vi "Ref Rectangle Selection Window.vi"(8 "error in (no error)":errorcluster) -> (0 "error out":errorcluster, 1 "Error or cancelled":bool)   [LabVIEW 2020]
uses:
  <vilib>/vision/Image Controls.llb/IMAQ Image.ctl
  Typedefs/Channel Selector.ctl
  Typedefs/Ref select window ctrl refs.ctl
  Typedefs/Save-Load enum.ctl
  <vilib>/Utility/miscctls.llb/LVPointTypeDef.ctl
  Globals/gl_Windows Ctrl refs.vi
  Movement Correction/Globals/gl_Movement correction globals.vi
  Global Variables/General Globals.vi
  Global Variables/gl_Images.vi
  Global Variables/gl_UI Ctrl Refs.vi
panel:
  in  "Auto \ncentering\nZ":bool
  in  "Z Ignore":u8=2
  in  "Z Lines":u8=5
  in  "Z pixels":i32=1
  in  "Z Step":i8=2
  out "Ref size":string
  out "Info message":string="Please close this window and run the live imaging mode first to acquire an image"
  out "Tool":i32(ring) items=["None", "Selection Tool", "Point Tool", "Line Tool", "Rectangle Tool", "Oval Tool", "Polygon Tool", "ClosedFreehandTool", "Annulus Tool", "Rotated Rectangle Tool", "Zoom Tool", "Pan Tool", "Polyline Tool", "Freehand Tool"]
  in  "Cancel":bool
  in  "Image intensity":cluster{i16, i16}(slide)={0, 4095} caption="Threshold" scale=0.0..4095.0
  in  "Channel Selector":T1=enum."Green Channel"
  out "AOL Z":dbl format="%#_g um"
  out "AOL Z-Planes":dbl[](array[numeric])
  out "Reference Rectangles":i16[][](array[numeric])
  in  "Full Frame":T2(plugin-control)
  out "Motor Z planes":dbl[](array[numeric])
  out "# of Planes":i32
  out "GreenImageArray":T2[](array[typedef])
  out "RedImageArray":T2[](array[typedef])
  in  "Boundary":i16=2
  in  "OK":bool
  out "Motor Z":dbl format="%#_g um"
  out "Z-Plane":i32 format="Plane %.0f"
  out "Threshold":i16[](array[numeric])
  out "Selected Rectangle":i16[](array[numeric])
  in  "Z-Plane Selector":i32(c297)=7 caption="Z-Plane"
  out "Selection Frame":T2(plugin-control)
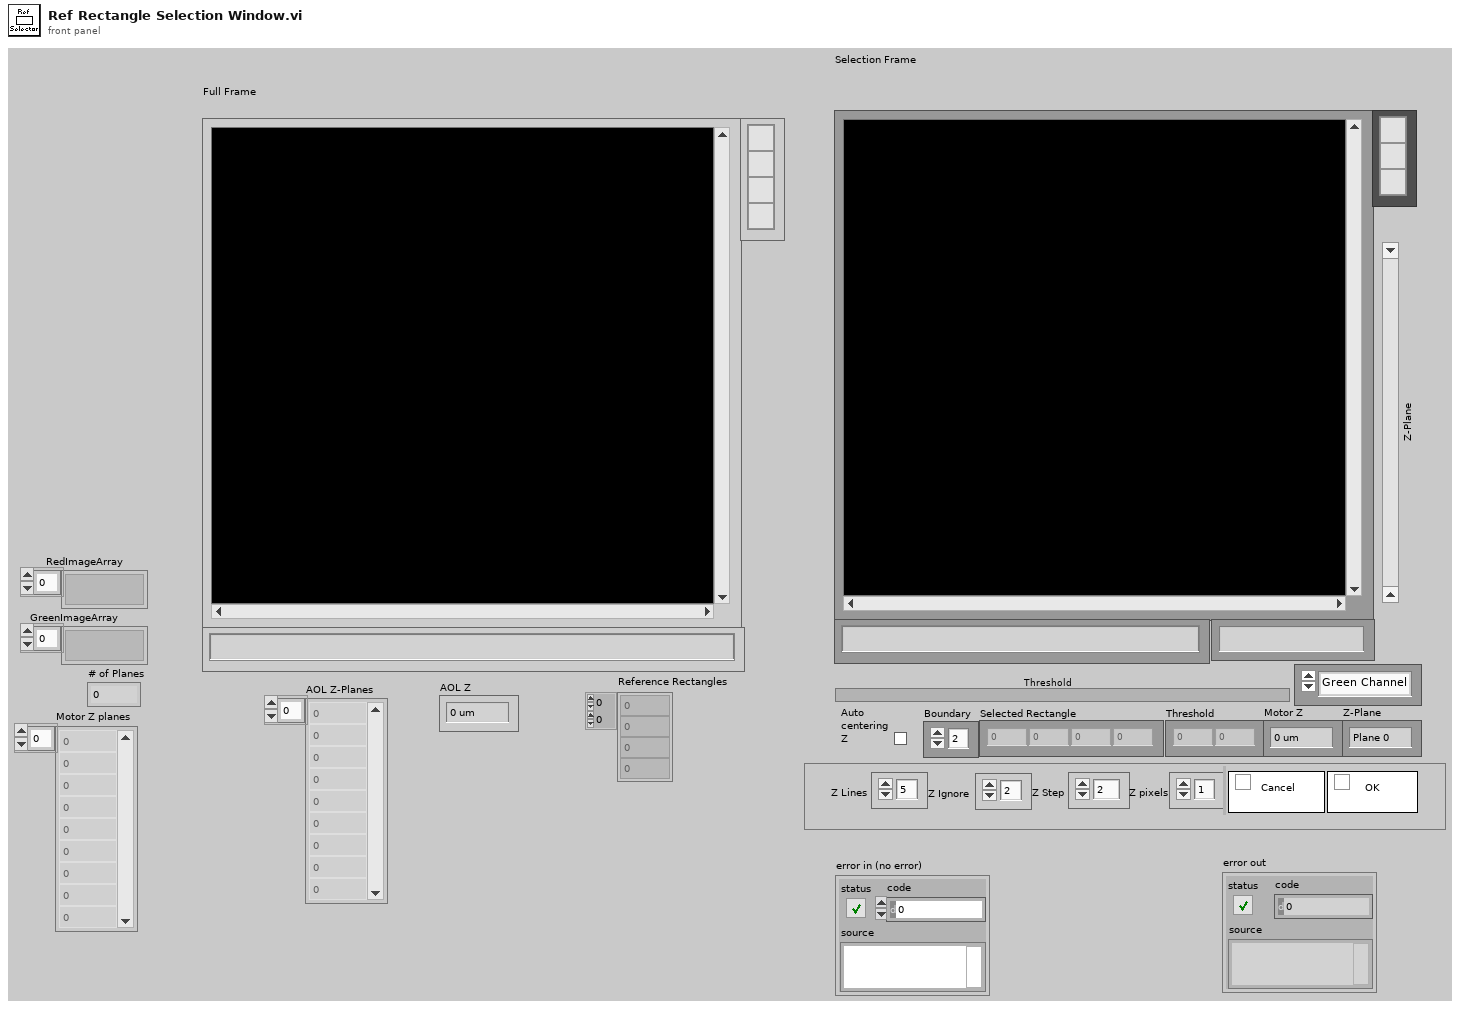
[diagram p1: front panel]
types:
  T1 = typedef "Channel Selector.ctl" = enum16{"Red Channel", "Green Channel", "Blended"}
  T2 = typedef "IMAQ Image.ctl" = refnum<image>
  T3 = typedef "Ref select window ctrl refs.ctl" = cluster{"Channel Selector":refnum<vi>, "Boundary":refnum<vi>, "Image intensity":refnum<vi>}
  T4 = typedef "Save-Load enum.ctl" = enum16{"Save to file", "Load from file", "Compare from file", "Save Backup"}
  T5 = enum16{"Show Binary", "Show Dendrite", "Find Lines"}
  T6 = typedef "LVPointTypeDef.ctl" = cluster{"Horizontal":i16, "Vertical":i16}
  T7 = cluster{"Conversion Method":u32, "Minimum Value":i32, "Maximum Value":i32, "Number Of Shifts":i32}
  T8 = typedef "Reference_Globals.ctl" = cluster{"Refrence data path":path, "Reference Rectangle":i16[][], "AOL Z":dbl, "No of pixels in a miniscan ":i32[], "Threshold":i16[], "No of miniscans":i32[], "Full Frame Size":u16, "Reference Image":T2, "dwelltime":dbl, "Zoom":dbl, "Field of View":dbl, "Z Step":i8, "Z pixels":i32, "Z Lines":u8, "Z Ignore":u8, "Laser":u8, "Auto centering":bool}
  T9 = typedef "AOL_Globals.ctl" = cluster{"Imaging Protocol":T10, "Number of POI":u16, "Number of Miniscans":u16, "Number of Trials":u16, "Number of Cycles ":u64, "# Averaged Frames":u16, "Laser power (%)":u8, "Pockels (V)":dbl, "Acquisition Length (sec)":dbl, "Fill time (us)":dbl, "POI Dwell time (us)":dbl, "Miniscan Dwell time per pixel (us)":dbl, "PMT 1":dbl, "PMT 2":dbl, "Back Apperture (mA)":dbl, "Frame Size":T11, "Center Frequency":dbl, "Field of View (norm)":dbl, "DwellTime (us)":dbl, "Wavelength (nm)":dbl, "Zoom":dbl, "AOL Z":dbl, "AOL Mode":T12, "GridXY":dbl, "GridZ":dbl, "TriggerPeriod (sec)":dbl, "Number of Pixels in Miniscan":u16, "Experiment folder path":path, "X centre":dbl, "Y centre":dbl, "Angle (degrees)":dbl, "Plane Mode":T13, "Threshold":u16[], "Regenerate Chirps":bool, "Rectangle ROI length (pixels)":u16, "Rectangle ROI height (pixels)":u16, "AOD fill":u16, "StartupDelay":i32, "Samples Wait after Trigger":u16, "Slip Cycle":u32, "Add Cycle":bool, "Functional Mode":T14, "Z Start":dbl, "Z Stop":dbl, "# Planes":i32, "Total Pixels":i32, "Variable Miniscan Pixels":u16[], "Use Variable Length":bool, "Use Variable Resolution":bool, "Laser power (%) at Z Start":u8, "Laser power (%) at Z Stop":u8, "Ref Z Step":i8, "Ref Dwell Time (us)":dbl, "Field of View (um)":dbl}
  T10 = typedef "Imaging Protocols enum.ctl" = enum16{"AOL Z-Stack", "Motor Z Stack", "Functional Acquisition", "Single Plane Acquisition", "Volume Acquisition", "Live Imaging", "Live Plane Imaging", "Live Volume Imaging"}
  T11 = typedef "Frame Size.ctl" = u16
  T12 = typedef "AOL modes.ctl" = enum16{"Raster", "Structural", "Pointing", "Mini Scan", "Alignment"}
  T13 = typedef "Plane Mode.ctl" = u16
  T14 = typedef "Functional Mode.ctl" = enum16{"Point", "Line", "Patch", "Plane", "Volume"}
  T15 = typedef "Ref DAQ Param.ctl" = cluster{"Full Frame Size":u16, "Ref Field of View":sgl, "Ref Zoom":i8, "Ref_dwellTime":sgl, "Ref X-pixels-per-line(Npxr)":i16, "Ref Y-lines-per-image(Npyr)":i16, "Ref Z-lines-per-image":i16, "Ignore Z lines":i16, "Ref Scan Cycles":i32, "Ref threshold XY":u16, "Ref threshold Z":u16, "Ref average XY":u16, "Ref Average  Z":u16, "Proportional_scale":fxp<+,16,2>, "Integral_scale":fxp<+/-,16,12>, "Proportional_scale Z":fxp<+,16,2>, "Integral_scale Z":fxp<+/-,16,12>, "Diff_threshold":fxp<+,16,2>, "Diff_threshold _z":fxp<+,16,2>, "Sliding Average":bool, "Ref count reset enabled":bool, "Auto-centering":bool}
  T16 = typedef "UI ctrl refs cluster.ctl" = cluster{"Top level VI path":path, "Top level VI ref":refnum<vi>, "User menu ref":refnum<k9>, "Sub Panel control":refnum<vi>, "Imaging Param Tab":refnum<vi>, "Occurrence-Start drivers":refnum<k4>, "Occurrence-Speed logging initialised":refnum<k4>, "Occurrence-XYZ stage initialised":refnum<k4>, "Exit button":refnum<vi>, "Status ind":refnum<vi>, "Set as origin":refnum<vi>, "Speed Logging":refnum<vi>, "Time Lapse":refnum<vi>, "Live Imaging":refnum<vi>, "AOL Z Stack":refnum<vi>, "Motor Z Stack":refnum<vi>, "Funct Acq button":refnum<vi>, "Hard Shutter":refnum<vi>, "Virtual Shutter":refnum<vi>, "Laser Power":refnum<vi>, "AOL Mode":refnum<vi>, "Frame Size":refnum<vi>, "Field of View":refnum<vi>, "Dwell Time":refnum<vi>, "Zoom":refnum<vi>, "AOL Z":refnum<vi>, "Objective":refnum<vi>, "Axis":refnum<vi>, "Paths & Names":refnum<vi>, "Experiment folder path (ind.)":refnum<vi>, "Last State (Ind.)":refnum<vi>, "Averages":refnum<vi>, "Angle (degrees)":refnum<vi>, "X centre":refnum<vi>, "Y centre":refnum<vi>, "Plane Mode":refnum<vi>, "# Planes":refnum<vi>, "Z Start":refnum<vi>, "Z Stop":refnum<vi>, "Z Step":refnum<vi>, "PMT 1":refnum<vi>, "PMT 2":refnum<vi>, "Stage XYZ Position":refnum<vi>, "Pockels@Z Start":refnum<vi>, "Pockels@Z Stop":refnum<vi>, "Obtain Z Start":refnum<vi>, "Obtain Z Stop":refnum<vi>, "Live stim.trig.period":refnum<vi>, "Live stim.trig.enable":refnum<vi>, "Movement Correction":refnum<vi>, "Load Reference Image":refnum<vi>, "XY Stage Move":refnum<vi>, "MovCor Cluster":refnum<vi>, "RefDAQParam":refnum<vi>, "Funct. Acq. Pockels Modulation":refnum<vi>, "Ref Laser Power":refnum<vi>, "Enable Video Recording":refnum<vi>, "Video Record-Live Imaging":refnum<vi>, "Video Record-Funct acq":refnum<vi>, "Reference Source":refnum<vi>, "AOL Z-stack Chirps Ready (ind)":refnum<vi>, "Target time between mov.cor. ref triggers (ms)":refnum<vi>, "Funct. Acq. Ref frame save":refnum<vi>, "Tracking button":refnum<vi>, "Show ref plots window":refnum<vi>, "Center freq ind (nm)":refnum<vi>, "Pickup mode (ind)":refnum<vi>, "Logging queue (ind)":refnum<vi>, "Back aperture power (ind.)":refnum<vi>, "Power after objective (ind.)":refnum<vi>, "Switch user":refnum<vi>, "Ls1 Conn. Status":refnum<vi>, "Ls1Tuning Status":refnum<vi>, "Ls1 Faults":refnum<vi>, "Ls1 Connection":refnum<vi>, "Ls1 Mode":refnum<vi>, "Ls1 POWER [mW]":refnum<vi>, "Ls1Shutter":refnum<vi>, "Ls1 Wavelength":refnum<vi>, "Ls1 Note":refnum<vi>, "Ls1 Confirm Wav":refnum<vi>, "Ls1 PreChrp Prism1":refnum<vi>, "Ls1 PreChrp Prism2":refnum<vi>, "Ls1 wav top Ind":refnum<vi>, "Ls1 power top Ind":refnum<vi>, "Ls1 Pump peak Hold":refnum<vi>, "Ls1 Status Ind":refnum<vi>, "Ls1 wav cancel":refnum<vi>, "Experiment Type":refnum<vi>, "Biology Information":refnum<vi>, "Camera recording status":refnum<vi>}
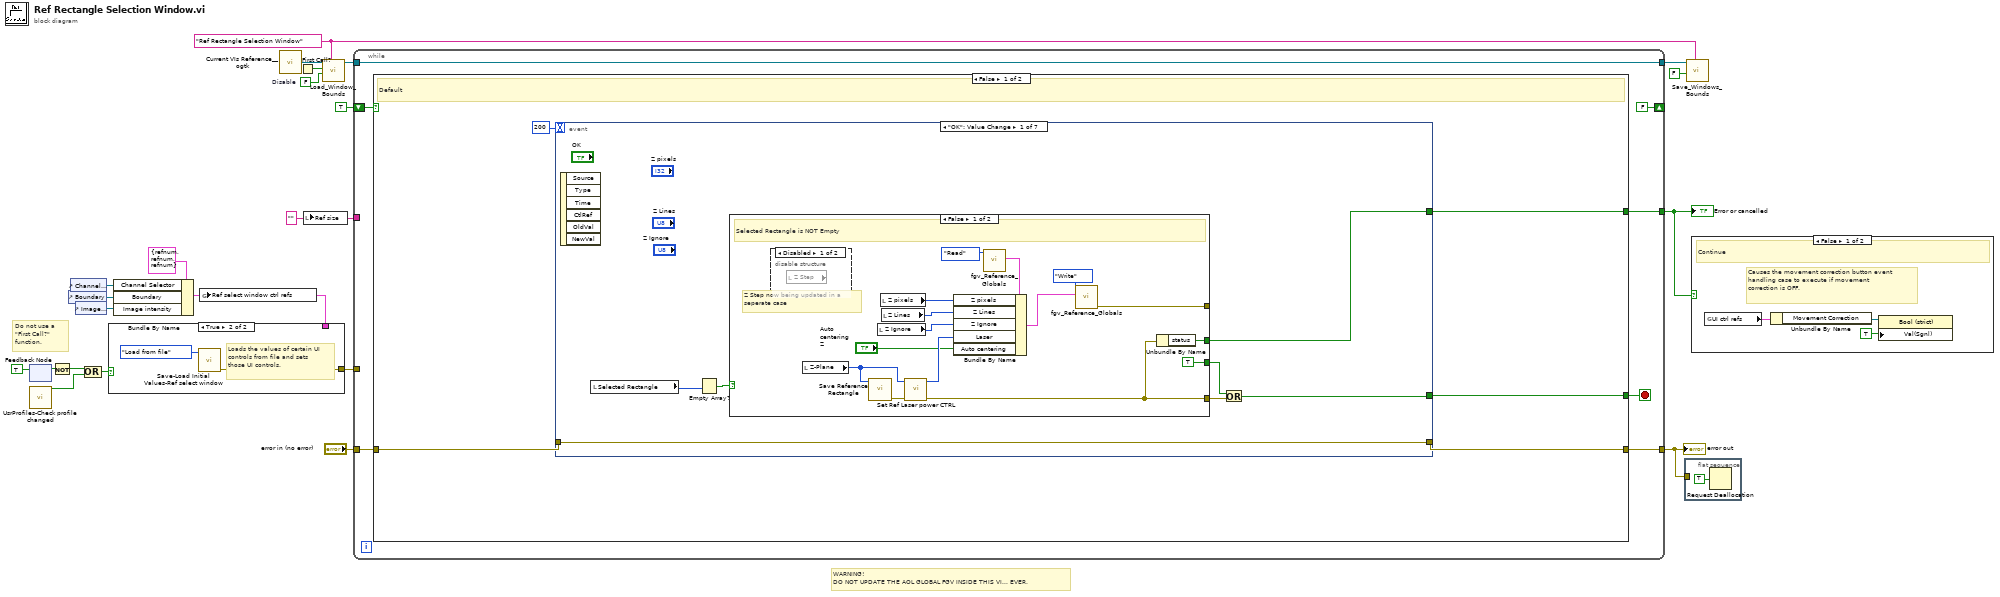
[diagram p0: block diagram]
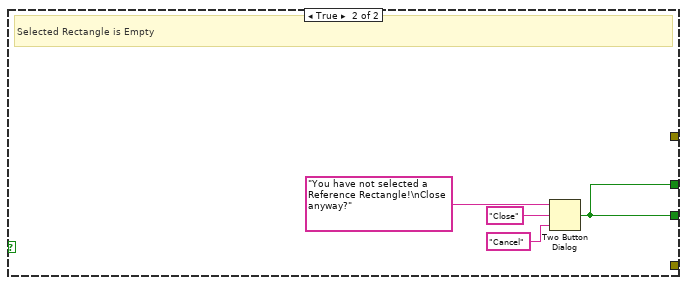
[diagram p5: hidden frame]
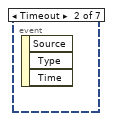
[diagram p6: hidden frame]
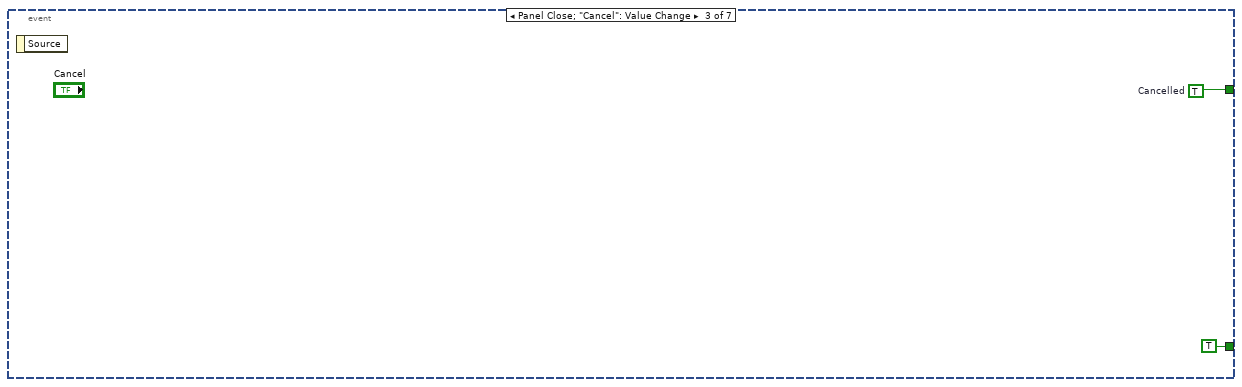
[diagram p7: hidden frame]
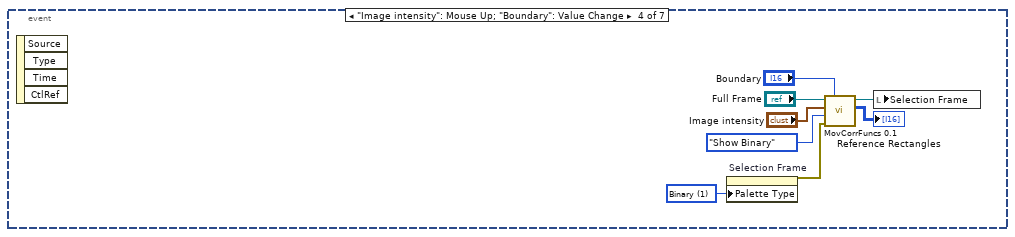
[diagram p8: hidden frame]
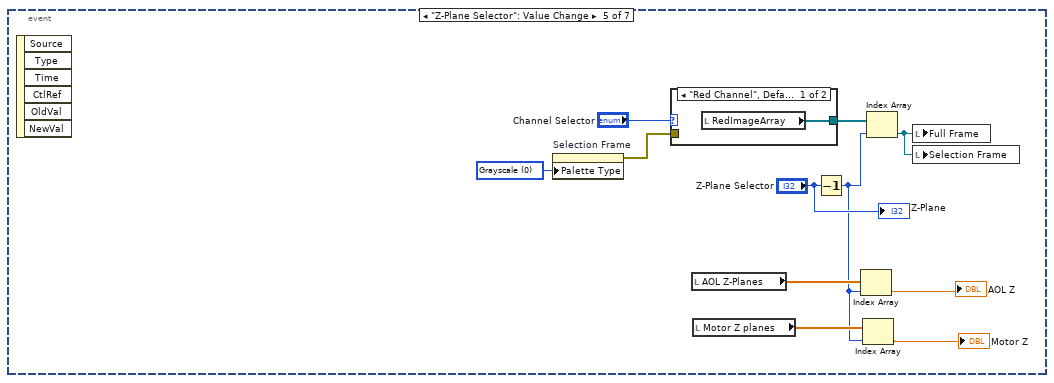
[diagram p9: hidden frame]
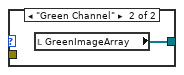
[diagram p10: hidden frame]
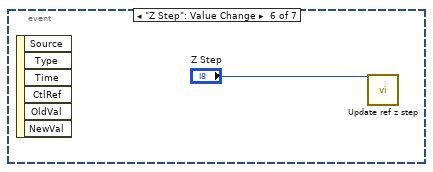
[diagram p11: hidden frame]
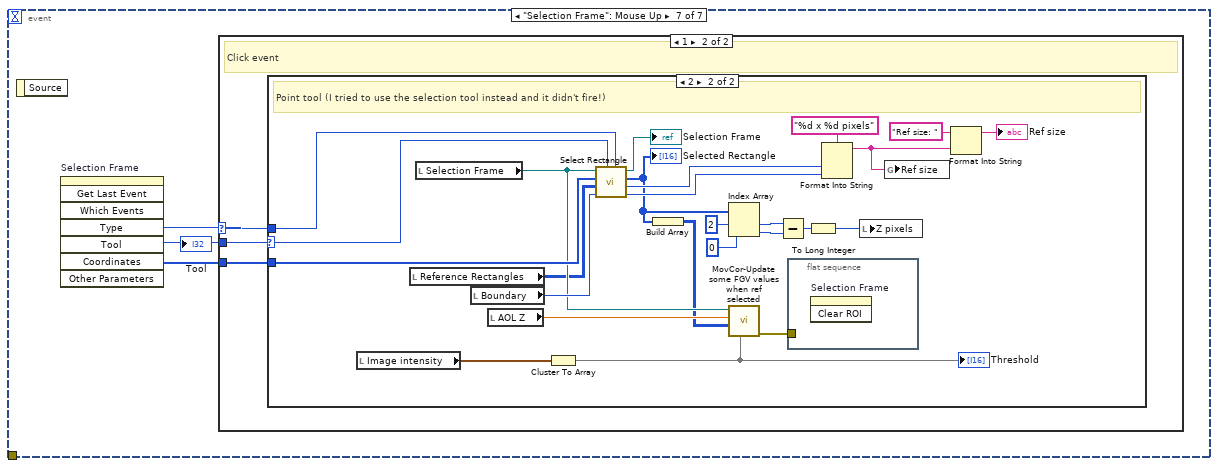
[diagram p12: hidden frame]
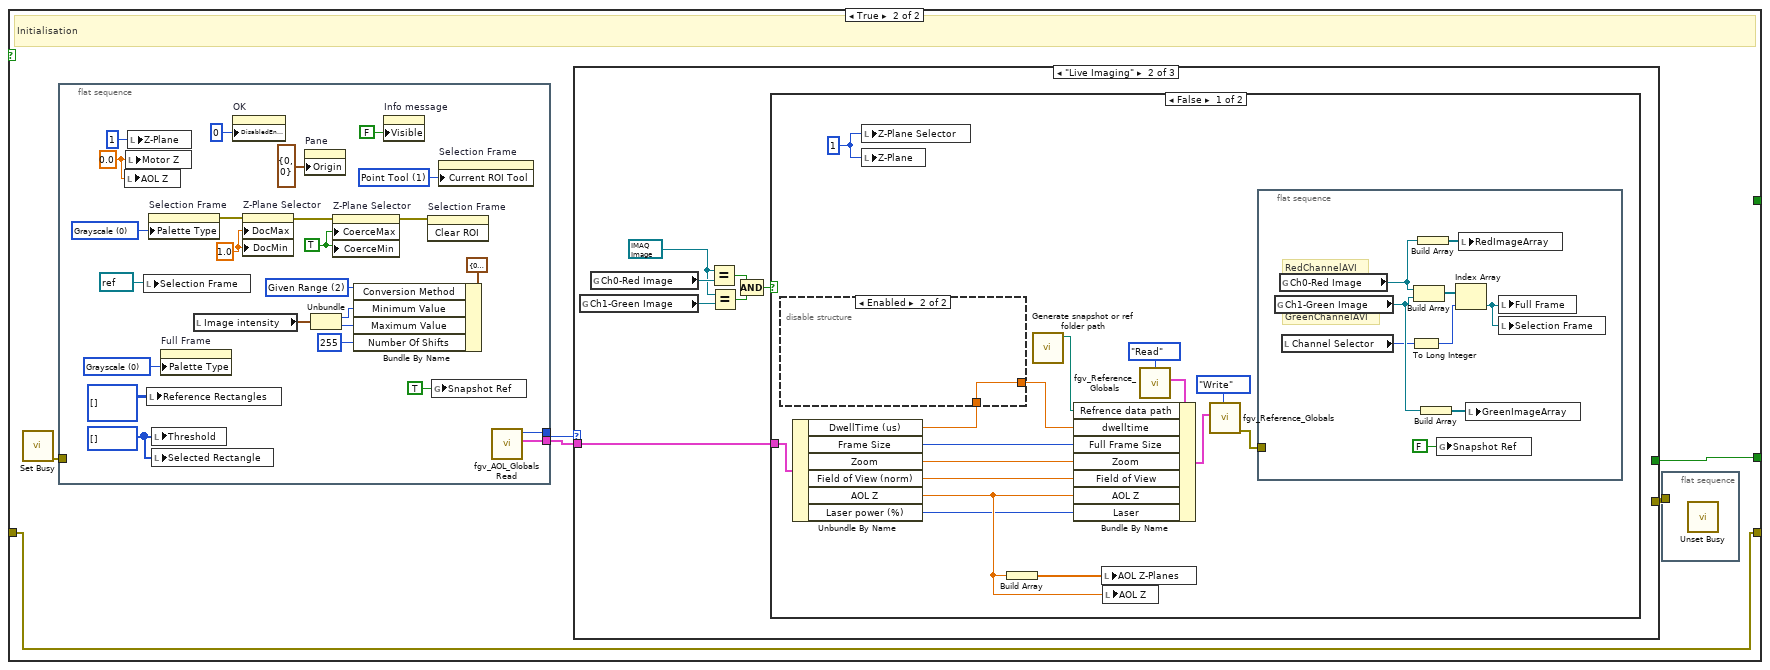
[diagram p15: hidden frame]
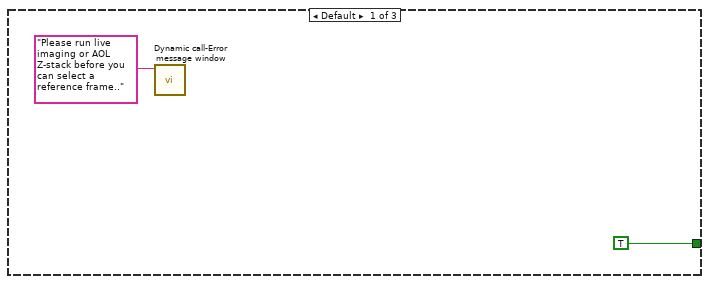
[diagram p16: hidden frame]
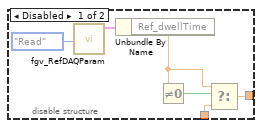
[diagram p17: hidden frame]
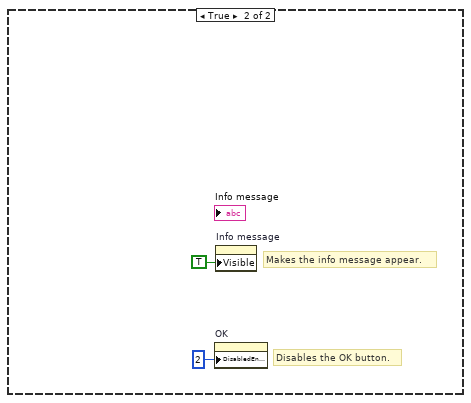
[diagram p18: hidden frame]
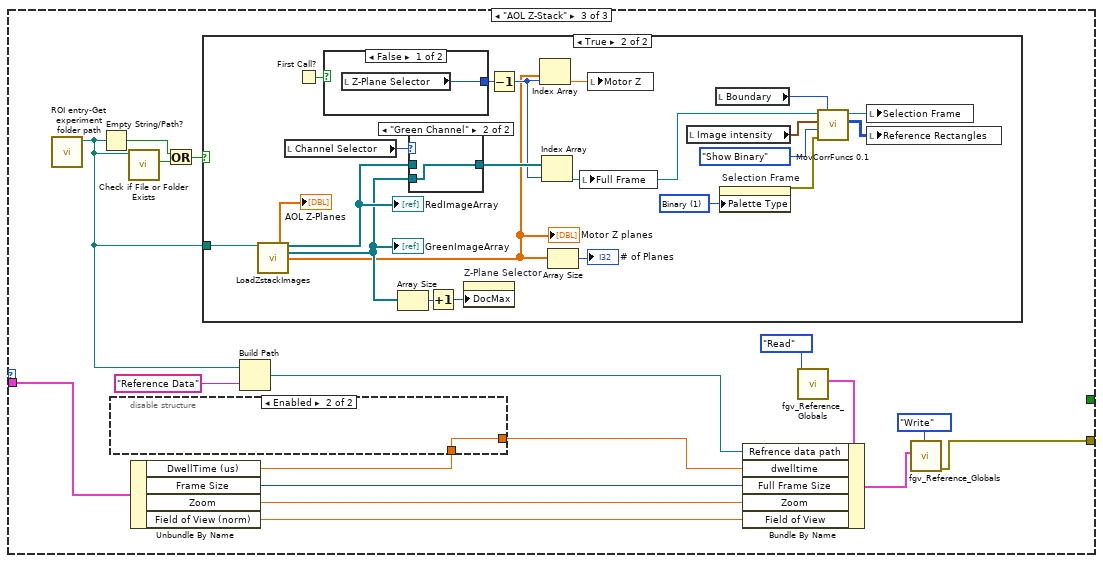
[diagram p19: hidden frame]
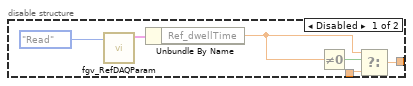
[diagram p20: hidden frame]
diagram:
  w13 = "" ("Ref size")
  w19 = FALSE  # Disable
  w15 = "Ref Rectangle Selection Window" ("Window Name (i.e. Key)")
  # "Do not use a \"First Call?\" function."
  # "WARNING!\nDO NOT UPDATE THE AOL GLOBAL FGV INSIDE THIS VI... EVER."
  n1 = feedback #1() -> (w5:bool)  [unwired: 1 in]
  n2 = feedback-in #1(TRUE) -> ()
  n3 = call "UsrProfiles-Check profile changed.vi"() -> ("Profile changed"=w2:bool)  [unwired: 10 in, 1 out]
  n4 = Not(x=w5) -> (.not. x?=w3:bool)
  n5 = control-ref of="Boundary"() -> (w10:refnum<vi>)
  n6 = control-ref of="Channel Selector"() -> (w11:refnum<vi>)
  n7 = control-ref of="Image intensity"() -> (w9:refnum<vi>)
  n8 = Compound Arithmetic op=OR(w3, w2) -> (w1:bool)
  n9 = Bundle By Name(cluster=T3 {"Channel Selector"=refnum, "Boundary"=refnum, "Image intensity"=refnum} ("Ref select window ctrl refs"), "Channel Selector"=w11, "Boundary"=w10, "Image intensity"=w9) -> (w7:T3)
  n10 = case shown="True" w1 {
    tunnel: [_ w24] -> w6
    tunnel: w7 -> [_ _]
    frame False {
    }
    frame True {
      # "Loads the values of certain UI controls from file and sets those UI controls."
      n11 = call "Save-Load Initial Values-Ref select window.vi"("Function"=Save-Load_enum."Load from file") -> ("error out"=w24:errorcluster)  [unwired: 10 in]
    }
  }
  n12 = global write "gl_Windows Ctrl refs.vi" "Ref select window ctrl refs"(w7) -> ()
  n13 = call <userlib>:"Current VIs Reference__ogtk.vi"() -> ("Current VI's reference"=w21:refnum<vi>)  [unwired: 5 in]
  n14 = First Call?() -> (First Call?: T/F=w20:bool)
  n15 = local write "Ref size"(w13) -> ()
  n16 = call "Load_Window_Bounds.vi"("Window Name (i.e. Key)"=w15, "Disable"=w19, "First Call"=w20, "Window VI's Ref"=w21) -> ("reference out"=w17:refnum<vi>)  [unwired: 4 in, 3 out]
  n17 = while {
    shift-right: [FALSE] -> _
    shift-left: TRUE -> [w30]
    tunnel: "error in (no error)" -> [w29]
    tunnel: [w28] -> w12
    tunnel: [w27] -> w14
    tunnel: [w26] -> w16
    tunnel: w17 -> [w26]
    tunnel: w13 -> [_]
    tunnel: w6 -> [_]
    stop <- w32 stop-if-true
    n18 = case shown="False" w30 {
      tunnel: [w36 w122] -> w32
      tunnel: w29 -> [w35 w119]
      tunnel: [w34 w119] -> w28
      tunnel: [w33 _] -> w27
      frame False {
        # "Default"
        n19 = event shown="[0] \"OK\": Value Change" {
          selector: _ -> [_ _ _ _ _ _ _]
          dyn-events: _ -> [_ _ _ _ _ _ _]
          timeout: 200 -> [_ _ _ _ _ _ _]
          tunnel: [w42 _ TRUE _ _ _ _] -> w36
          tunnel: w35 -> [w43 _ _ _ _ _ _]
          tunnel: [w43 _ _ _ _ _ _] -> w34
          tunnel: [w38 _ w64 _ _ _ _] -> w33
          event "OK": Value Change {
            n20 = event-data() -> ()  [unwired: 1 in, 6 out]
            n21 = local read "Selected Rectangle"() -> (w41:i16[])
            n22 = Empty Array?(array=w41) -> (empty?=w40:bool)
            n23 = case shown="False" w40 {
              tunnel: [TRUE ("T button?") w62] -> w39
              tunnel: [w55 _] -> w44
              tunnel: [w58 w62] -> w38
              tunnel: [w52 _] -> _
              frame False {
                # "Z Step now being updated in a\nseperate case"
                # "Selected Rectangle is NOT Empty"
                n24 = disable-structure shown="Disabled" {
                  frame Disabled {
                    n25 = local read "Z Step"() -> ()  [unwired: 1 out]
                  }
                  frame Enabled {
                  }
                }
                n26 = local read "Z-Plane"() -> (w56:i32)
                n27 = call "Save Reference Rectangle.vi"("Z-Plane"=w56) -> ("error out"=w57:errorcluster)  [unwired: 10 in]
                n28 = local read "Z Ignore"() -> (w46:u8)
                n29 = local read "Z pixels"() -> (w49:i32)
                n30 = local read "Z Lines"() -> (w48:u8)
                n31 = call "Set Ref Laser power CTRL.vi"("error in (no error)"=w57, "Z-Plane"=w56) -> ("error out"=w55:errorcluster, "Laser power (%)"=w47:u8)  [unwired: 8 in]
                n32 = call "fgv_Reference_Globals.vi"("Function"=enum16{"Intialize", "Write", "Read", "Clear"}."Read") -> ("Reference Data"=w50:T8)  [unwired: 9 in, 1 out]
                n33 = Bundle By Name(cluster=w50, "Z pixels"=w49, "Z Lines"=w48, "Z Ignore"=w46, "Laser"=w47, "Auto centering"="Auto \ncentering\nZ") -> (w51:T8)
                n34 = call "fgv_Reference_Globals.vi"("Reference Data"=w51, "Function"=enum16{"Intialize", "Write", "Read", "Clear"}."Write") -> ("error out"=w52:errorcluster)  [unwired: 8 in, 1 out]
                n35 = Unbundle By Name(w55) -> ("status"=w58:bool)
              }
              frame True {
                # "Selected Rectangle is Empty"
                n36 = Two Button Dialog(message="You have not selected a Reference Rectangle!\nClose anyway?", 1:"Cancel" ("F button name (\"Cancel\")"), 2:"Close" ("T button name (\"OK\")")) -> (T button?=w62:bool)
              }
            }
            n37 = Or(x=w39, y=w44) -> (x .or. y?=w42:bool)
          }
          event Timeout {
            n38 = event-data() -> ()  [unwired: 1 in, 3 out]
          }
          event Panel Close; "Cancel": Value Change {
            w64 = TRUE  # Cancelled
            n39 = event-data() -> ()  [unwired: 1 in, 1 out]
          }
          event "Image intensity": Mouse Up; "Boundary": Value Change {
            w68 = u32 1 items=["Grayscale", "Binary", "Gradient", "Rainbow", "Temperature", "User Defined"] ("Palette:Palette Type")
            n40 = event-data() -> ()  [unwired: 1 in, 4 out]
            n41 = property on="Selection Frame" class="ImageControl"("Palette Type"=w68) -> (error out=w69:errorcluster)  [unwired: 2 in, 1 out]
            n42 = call "MovCorrFuncs 0.1.vi"("Boundary"="Boundary", "error in (no error)"=w69, "MovCorrFunc"=T5."Show Binary" ("Move Corr Function"), "LUT1"="Image intensity", "Image"="Full Frame") -> ("Reference Rectangles"=→"Reference Rectangles":i16[][], "Reference Screen"=w73:T2)  [unwired: 4 in, 1 out]
            n43 = local write "Selection Frame"(w73) -> ()
          }
          event "Z-Plane Selector": Value Change {
            w82 = u32 0 items=["Grayscale", "Binary", "Gradient", "Rainbow", "Temperature", "User Defined"] ("Palette:Palette Type")
            n44 = event-data() -> ()  [unwired: 1 in, 6 out]
            n45 = property on="Selection Frame" class="ImageControl"("Palette Type"=w82) -> (error out=w81:errorcluster)  [unwired: 2 in, 1 out]
            n46 = case shown="\"Red Channel\", Default" "Channel Selector" {
              tunnel: [w85 w86] -> w84
              tunnel: w81 -> [_ _]
              frame "Red Channel", Default {
                n47 = local read "RedImageArray"() -> (w85:T2[])
              }
              frame "Green Channel" {
                n48 = local read "GreenImageArray"() -> (w86:T2[])
              }
            }
            n49 = local read "AOL Z-Planes"() -> (w76:dbl[])
            n50 = local read "Motor Z planes"() -> (w79:dbl[])
            n51 = Decrement(x="Z-Plane Selector") -> (x-1=w74:i32)
            n52 = Index Array(array=w76, index=w74) -> (element=→"AOL Z":dbl)
            n53 = Index Array(array=w79, index=w74) -> (element=→"Motor Z":dbl)
            n54 = Index Array(array=w84, index=w74) -> (element=w83:T2)
            n55 = local write "Full Frame"(w83) -> ()
            n56 = local write "Selection Frame"(w83) -> ()
            "Z-Plane" <- "Z-Plane Selector"
          }
          event "Z Step": Value Change {
            n57 = event-data() -> ()  [unwired: 1 in, 6 out]
            n58 = call "Update ref z step.vi"("Ref Z Step [µm]"="Z Step") -> ()  [unwired: 10 in, 1 out]
          }
          event "Selection Frame": Mouse Up {
            n59 = event-data() -> ()  [unwired: 1 in, 1 out]
            n60 = invoke on="Selection Frame" class="ImageControl" method="Get Last Event"() -> ("Type"=w90:i32, "Tool"=w89:i32, "Coordinates"=w88:i32[])  [unwired: 8 in, 5 out]
            "Tool" <- w89
            n61 = case shown="1" w90 {
              selector: w90 -> [_ w92]
              tunnel: w89 -> [_ w91]
              tunnel: w88 -> [_ w93]
              frame Default {
                # "Any other event"
              }
              frame 1 {
                # "Click event"
                n62 = case shown="2" w91 {
                  selector: w91 -> [_ w113]
                  tunnel: w93 -> [_ w118]
                  tunnel: w92 -> [_ w117]
                  frame Default {
                    # "Any other tool"
                  }
                  frame 2 {
                    # "Point tool (I tried to use the selection tool instead and it didn't fire!)"
                    n63 = local read "Image intensity"() -> (w116:cluster{i16, i16})
                    n64 = local read "Reference Rectangles"() -> (w104:i16[][])
                    n65 = local read "Selection Frame"() -> (w106:T2)
                    n66 = local read "Boundary"() -> (w115:i16)
                    n67 = local read "AOL Z"() -> (w105:dbl)
                    n68 = Cluster To Array(cluster=w116) -> (array=w103:i16[])
                    "Threshold" <- w103
                    n69 = call "Select Rectangle.vi"("Type"=w117, "Tool"=w113, "Boundary"=w115, "Reference Rectangle"=w104, "Coordinates"=w118, "Image In"=w106) -> ("Height (pixels)"=w110:i32, "Width (pixels)"=w111:i32, "Selected Reference Rectangle"=w100:i16[], "Image Out"=→"Selection Frame":T2)  [unwired: 2 in]
                    "Selected Rectangle" <- w100
                    n70 = Build Array(w100) -> (w101:i16[][])
                    n71 = Index Array(array=w100, index #1=2 ("index"), index #2=0 ("index")) -> (element #1=w96:i16, element #2=w97:i16)
                    n72 = call "MovCor-Update some FGV values when ref selected.vi"("Threshold"=w103, "Reference Rectangles"=w101, "AOL Z"=w105, "Reference image"=w106) -> ("error out"=w102:errorcluster)  [unwired: 7 in]
                    n73 = Subtract(x=w96, y=w97) -> (x-y=w95:i16)
                    n74 = flat-sequence {
                      tunnel: w102 -> [_]
                      frame #0 {
                        n75 = invoke on="Selection Frame" class="ImageControl" method="Clear ROI"() -> ()  [unwired: 3 in, 3 out]
                      }
                    }
                    n76 = To Long Integer(number=w95) -> (32bit integer=w94:i32)
                    n77 = Format Into String(format string="%d x %d pixels", w111, w110) -> (resulting string=w107:string)  [unwired: 2 in, 1 out]
                    n78 = local write "Z pixels"(w94) -> ()
                    n79 = global write "gl_Movement correction globals.vi" "Ref size"(w107) -> ()
                    n80 = Format Into String(initial string="Ref size: " ("format string"), w107) -> (resulting string=→"Ref size":string)  [unwired: 2 in, 1 out]
                  }
                }
              }
            }
          }
        }
      }
      frame True {
        # "Initialisation"
        n81 = call <vilib>:"Set Busy.vi"() -> ("error out"=w120:errorcluster)  [unwired: 10 in, 1 out]
        n82 = flat-sequence {
          tunnel: [w125] -> w124
          tunnel: [w126] -> w123
          tunnel: w120 -> [_]
          frame #0 {
            w130 = u32 1 items=["Zoom Tool"=8, "Selection Tool"=0, "Pan Tool"=9, "Point Tool"=1, "Line Tool"=2, "Rectangle Tool"=3, "Rotated Rectangle Tool"=12, "Polyline Tool"=10, "Polygon Tool"=5, "Freehand Tool"=11, "Closed Freehand Tool"=6, "Ellipse Tool"=4, "Annulus Tool"=7] ("Current ROI Tool")
            w133 = 0.0 ("Motor Z")
            w127 = i16[] [] ("Threshold")
            w136 = u32 0 items=["Grayscale", "Binary", "Gradient", "Rainbow", "Temperature", "User Defined"] ("Palette:Palette Type")
            w140 = u32 2 items=["Full Dynamic", "Downshift", "Given Range", "90 % Dynamic", "Given Percent Range"] ("Conversion Method")
            w146 = TRUE ("Coerce Maximum Value")
            w148 = 1.0 ("Doc Min")
            w149 = u32 0 items=["Grayscale", "Binary", "Gradient", "Rainbow", "Temperature", "User Defined"] ("Palette:Palette Type")
            n83 = local write "AOL Z"(w133) -> ()
            n84 = local write "Motor Z"(w133) -> ()
            n85 = local write "Z-Plane"(1 ("Z-Plane")) -> ()
            n86 = local write "Selection Frame"(refnum<image> refnum ("Zstack")) -> ()
            n87 = local write "Reference Rectangles"(i16[][] [] ("Reference Rectangles")) -> ()
            n88 = property on="Selection Frame" class="ImageControl"("Palette Type"=w149) -> (error out=w147:errorcluster)  [unwired: 2 in, 1 out]
            n89 = local write "Threshold"(w127) -> ()
            n90 = local write "Selected Rectangle"(w127) -> ()
            n91 = property on="Full Frame" class="ImageControl"("Palette Type"=w136) -> ()  [unwired: 2 in, 2 out]
            n92 = local read "Image intensity"() -> (w137:cluster{i16, i16})
            n93 = property on="OK" class="Bool"("DisabledEnum"=0) -> ()  [unwired: 2 in, 2 out]
            n94 = property on="Z-Plane Selector" class="Scroll (strict)"(error in=w147, "DocMax"=w148, "DocMin"=w148) -> (error out=w145:errorcluster)  [unwired: 1 in, 1 out]
            n95 = property on="Pane" class="Pane"("Origin"=T6 {"Horizontal"=0, "Vertical"=0}) -> ()  [unwired: 2 in, 2 out]
            n96 = Unbundle(w137) -> (w142:i16, w141:i16)
            n97 = property on="Z-Plane Selector" class="Scroll (strict)"(error in=w145, "CoerceMax"=w146, "CoerceMin"=w146) -> (error out=w143:errorcluster)  [unwired: 1 in, 1 out]
            n98 = Bundle By Name(cluster=T7 {"Conversion Method"=0, "Minimum Value"=0, "Maximum Value"=0, "Number Of Shifts"=0} ("16-bit Display Mapping:All Elements"), "Conversion Method"=w140, "Minimum Value"=w142, "Maximum Value"=w141, "Number Of Shifts"=255) -> ()  [unwired: 1 out]
            n99 = property on="Info message" class="Str"("Visible"=FALSE) -> ()  [unwired: 2 in, 2 out]
            n100 = invoke on="Selection Frame" class="ImageControl" method="Clear ROI"(error in=w143) -> ()  [unwired: 2 in, 3 out]
            n101 = global write "General Globals.vi" "Snapshot Ref"(TRUE ("Snapshot Ref")) -> ()
            n102 = property on="Selection Frame" class="ImageControl"("Current ROI Tool"=w130) -> ()  [unwired: 2 in, 2 out]
            n103 = call "fgv_AOL_Globals Read.vi"() -> ("AOL_Globals"=w126:T9, "Imaging Protocol"=w125:T10)  [unwired: 9 in, 1 out]
          }
        }
        n104 = case shown="\"Live Imaging\"" w124 {
          tunnel: [_ _ w203] -> w121
          tunnel: w123 -> [_ w158 w200]
          tunnel: [TRUE _ _] -> w122
          frame Default {
            n105 = call "Dynamic call-Error message window.vi"("Error Message"="Please run live imaging or AOL Z-stack before you can select a reference frame..") -> ()  [unwired: 10 in, 1 out]
          }
          frame "Live Imaging" {
            w156 = T2 refnum ("Ref Ch0 Image")
            n106 = global read "gl_Images.vi" "Ch1-Green Image"() -> (w155:T2)
            n107 = global read "gl_Images.vi" "Ch0-Red Image"() -> (w157:T2)
            n108 = Equal?(x=w156, y=w157) -> (x = y?=w154:bool)
            n109 = Equal?(x=w156, y=w155) -> (x = y?=w153:bool)
            n110 = Compound Arithmetic op=AND(w154, w153) -> (w152:bool)
            n111 = case shown="False" w152 {
              tunnel: w158 -> [w171 _]
              frame False {
                w166 = 1 ("Z-Plane Selector")
                n112 = Unbundle By Name(w171) -> ("DwellTime (us)"=w160:dbl, "Frame Size"=w170:T11, "Zoom"=w169:dbl, "Field of View (norm)"=w163:dbl, "AOL Z"=w164:dbl, "Laser power (%)"=w162:u8)
                n113 = disable-structure shown="Enabled" {
                  disable-tunnel: w160 -> [w176 w181]
                  disable-tunnel: [w175 w181] -> w159
                  frame Disabled {
                    n114 = call "fgv_RefDAQParam.vi"("Function"=enum16{"Initialize", "Write", "Read"}."Read" ("Status")) -> ("RefDAQParam"=w179:T15)  [unwired: 9 in, 1 out]
                    n115 = Unbundle By Name(w179) -> ("Ref_dwellTime"=w177:sgl)
                    n116 = Not Equal To 0?(x=w177) -> (x != 0?=w178:bool)
                    n117 = Select(t=w177, s=w178, f=w176) -> (s? t:f=w175:dbl)
                  }
                  frame Enabled {
                  }
                }
                n118 = local write "Z-Plane Selector"(w166) -> ()
                n119 = local write "Z-Plane"(w166) -> ()
                n120 = Build Array(w164) -> (w168:dbl[])
                n121 = call "Generate snapshot or ref folder path.vi"() -> ("Snapshot folder path"=w161:path)  [unwired: 10 in, 1 out]
                n122 = local write "AOL Z-Planes"(w168) -> ()
                n123 = local write "AOL Z"(w164) -> ()
                n124 = call "fgv_Reference_Globals.vi"("Function"=enum16{"Intialize", "Write", "Read", "Clear"}."Read") -> ("Reference Data"=w173:T8)  [unwired: 9 in, 1 out]
                n125 = Bundle By Name(cluster=w173, "Refrence data path"=w161, "dwelltime"=w159, "Full Frame Size"=w170, "Zoom"=w169, "Field of View"=w163, "AOL Z"=w164, "Laser"=w162) -> (w165:T8)
                n126 = call "fgv_Reference_Globals.vi"("Reference Data"=w165, "Function"=enum16{"Intialize", "Write", "Read", "Clear"}."Write") -> ("error out"=w167:errorcluster)  [unwired: 8 in, 1 out]
                n127 = flat-sequence {
                  tunnel: w167 -> [_]
                  frame #0 {
                    # "GreenChannelAVI"
                    # "RedChannelAVI"
                    n128 = global read "gl_Images.vi" "Ch1-Green Image"() -> (w187:T2)
                    n129 = global read "gl_Images.vi" "Ch0-Red Image"() -> (w188:T2)
                    n130 = local read "Channel Selector"() -> (w183:T1)
                    n131 = To Long Integer(number=w183) -> (32bit integer=w182:i32)
                    n132 = Build Array(w188, w187) -> (w190:T2[])
                    n133 = Build Array(w188) -> (w189:T2[])
                    n134 = Build Array(w187) -> (w186:T2[])
                    n135 = global write "General Globals.vi" "Snapshot Ref"(FALSE ("Snapshot Ref")) -> ()
                    n136 = Index Array(array=w190, index=w182) -> (element=w185:T2)
                    n137 = local write "RedImageArray"(w189) -> ()
                    n138 = local write "GreenImageArray"(w186) -> ()
                    n139 = local write "Full Frame"(w185) -> ()
                    n140 = local write "Selection Frame"(w185) -> ()
                  }
                }
              }
              frame True {
                # "Makes the info message appear."
                # "Disables the OK button."
                n141 = property on="OK" class="Bool"("DisabledEnum"=2) -> ()  [unwired: 2 in, 2 out]
                n142 = property on="Info message" class="Str"("Visible"=TRUE) -> ()  [unwired: 2 in, 2 out]
              }
            }
          }
          frame "AOL Z-Stack" {
            n143 = call "ROI entry-Get experiment folder path.vi"() -> ("Experiment folder path"=w196:path)  [unwired: 10 in, 1 out]
            n144 = Empty String/Path?(string/path=w196) -> (empty?=w209:bool)
            n145 = call <vilib>:"Check if File or Folder Exists.vi"("path"=w196) -> ("file or folder exists?"=w207:bool)  [unwired: 8 in, 2 out]
            n146 = Unbundle By Name(w200) -> ("DwellTime (us)"=w194:dbl, "Frame Size"=w202:T11, "Zoom"=w201:dbl, "Field of View (norm)"=w197:dbl)
            n147 = disable-structure shown="Enabled" {
              disable-tunnel: w194 -> [w211 w216]
              disable-tunnel: [w210 w216] -> w193
              frame Disabled {
                n148 = call "fgv_RefDAQParam.vi"("Function"=enum16{"Initialize", "Write", "Read"}."Read" ("Status")) -> ("RefDAQParam"=w214:T15)  [unwired: 9 in, 1 out]
                n149 = Unbundle By Name(w214) -> ("Ref_dwellTime"=w212:sgl)
                n150 = Not Equal To 0?(x=w212) -> (x != 0?=w213:bool)
                n151 = Select(t=w212, s=w213, f=w211) -> (s? t:f=w210:dbl)
              }
              frame Enabled {
              }
            }
            n152 = Or(x=w209, y=w207) -> (x .or. y?=w208:bool)
            n153 = case shown="True" w208 {
              tunnel: w196 -> [_ w238]
              frame False {
              }
              frame True {
                w219 = u32 1 items=["Grayscale", "Binary", "Gradient", "Rainbow", "Temperature", "User Defined"] ("Palette:Palette Type")
                n154 = call "LoadZstackImages.vi"("Experiment folder path OR Z-stack folder path"=w238) -> ("AOL Z Planes"=→"AOL Z-Planes":dbl[], "Red Image Array"=w231:T2[], "Green Image Array"=w230:T2[], "Motor Z planes"=w229:dbl[])  [unwired: 5 in, 6 out]
                "RedImageArray" <- w231
                "GreenImageArray" <- w230
                "Motor Z planes" <- w229
                n155 = local read "Channel Selector"() -> (w226:T1)
                n156 = First Call?() -> (First Call?: T/F=w234:bool)
                n157 = case shown="False" w234 {
                  tunnel: [w239 w240] -> w232
                  frame False {
                    n158 = local read "Z-Plane Selector"() -> (w239:i32)
                  }
                  frame True {
                    w240 = 1 ("Z-Plane Selector")
                    n159 = local write "Z-Plane Selector"(w240) -> ()
                    n160 = local write "Z-Plane"(w240) -> ()
                  }
                }
                n161 = Array Size(array=w230) -> (size(s)=w237:i32)
                n162 = case shown="\"Green Channel\"" w226 {
                  tunnel: [w241 w242] -> w235
                  tunnel: w231 -> [w241 _]
                  tunnel: w230 -> [_ w242]
                  frame "Red Channel", Default {
                  }
                  frame "Green Channel" {
                  }
                }
                n163 = Increment(x=w237) -> (x+1=w236:i32)
                n164 = property on="Z-Plane Selector" class="Scroll (strict)"("DocMax"=w236) -> ()  [unwired: 2 in, 2 out]
                n165 = Decrement(x=w232) -> (x-1=w233:i32)
                n166 = Index Array(array=w229, index=w233) -> (element=w227:dbl)
                n167 = Index Array(array=w235, index=w233) -> (element=w218:T2)
                n168 = Array Size(array=w229) -> (size(s)=→"# of Planes":i32)
                n169 = local write "Full Frame"(w218) -> ()
                n170 = local write "Motor Z"(w227) -> ()
                n171 = local read "Image intensity"() -> (w224:cluster{i16, i16})
                n172 = local read "Boundary"() -> (w223:i16)
                n173 = property on="Selection Frame" class="ImageControl"("Palette Type"=w219) -> (error out=w220:errorcluster)  [unwired: 2 in, 1 out]
                n174 = call "MovCorrFuncs 0.1.vi"("Boundary"=w223, "error in (no error)"=w220, "MovCorrFunc"=T5."Show Binary" ("Move Corr Function"), "LUT1"=w224, "Image"=w218) -> ("Reference Rectangles"=w225:i16[][], "Reference Screen"=w222:T2)  [unwired: 4 in, 1 out]
                n175 = local write "Selection Frame"(w222) -> ()
                n176 = local write "Reference Rectangles"(w225) -> ()
              }
            }
            n177 = Build Path(base path=w196, name or relative path="Reference Data") -> (appended path=w195:path)
            n178 = call "fgv_Reference_Globals.vi"("Function"=enum16{"Intialize", "Write", "Read", "Clear"}."Read") -> ("Reference Data"=w199:T8)  [unwired: 9 in, 1 out]
            n179 = Bundle By Name(cluster=w199, "Refrence data path"=w195, "dwelltime"=w193, "Full Frame Size"=w202, "Zoom"=w201, "Field of View"=w197) -> (w198:T8)
            n180 = call "fgv_Reference_Globals.vi"("Reference Data"=w198, "Function"=enum16{"Intialize", "Write", "Read", "Clear"}."Write") -> ("error out"=w203:errorcluster)  [unwired: 8 in, 1 out]
          }
        }
        n181 = flat-sequence {
          tunnel: w121 -> [_]
          frame #0 {
            n182 = call <vilib>:"Unset Busy.vi"() -> ()  [unwired: 11 in, 1 out]
          }
        }
      }
    }
  }
  "error out" <- w12
  "Error or cancelled" <- w14
  n183 = flat-sequence {
    tunnel: w12 -> [_]
    frame #0 {
      n184 = Request Deallocation(TRUE ("flag")) -> ()
    }
  }
  n185 = call "Save_Windows_Bounds.vi"("Window Name (i.e. Key)"=w15, "Front Panel Window:Open"=FALSE, "Window VI's Ref"=w16) -> ()  [unwired: 8 in, 1 out]
  n186 = case shown="False" w14 {
    frame False {
      # "Causes the movement correction button event handling case to execute if movement correction is OFF."
      # "Continue"
      n187 = global read "gl_UI Ctrl Refs.vi" "UI ctrl refs"() -> (w244:T16)
      n188 = Unbundle By Name(w244) -> ("Movement Correction"=w246:refnum<vi>)
      n189 = property on="Property Node" class="Bool (strict)"(reference=w246, "Val(Sgnl)"=TRUE ("Movement Correction ON?")) -> ()  [unwired: 1 in, 2 out]
    }
    frame True {
      # "Cancelled"
    }
  }
